vi "Set Multi.vi"(0 "Display State In":T2, 5 "Value":T1={"Active"=FALSE, "Delay (ms)"=0.0, "Duration (ms)"=50.0, "Ramp (ms)"=5.0, "Rate (Hz)"=0.0, "Trepeat (ms)"=0.0, "Repeat"=FALSE}, 7 "First":bool, 9 "Container State":T3, 11 "error in (no error)":errorcluster) -> (4 "Display State Out":T2, 15 "error out":errorcluster)   [LabVIEW 2015, in "Burst (G3).xctl"]
uses:
  Burst (G3).xctl
  <vilib>/_xctls/Container State.ctl
  State.ctl
  Utility VIs/Controls/KCheckbox/KCheckbox.xctl
  Utility VIs/Controls/KNumeric (DBL)/KNumeric (DBL).xctl
  Burst Data.ctl
  <vilib>/_xctls/XControlSupport.lvlib
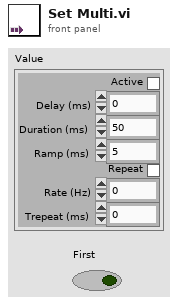
[diagram p1: front panel]
types:
  T1 = typedef "Burst (G3).xctl/Burst Data.ctl" = cluster{"Active":bool, "Delay (ms)":dbl, "Duration (ms)":dbl, "Ramp (ms)":dbl, "Rate (Hz)":dbl, "Trepeat (ms)":dbl, "Repeat":bool}
  T2 = typedef "Burst (G3).xctl/State.ctl" = cluster{"ctls":cluster{"Active":refnum<vi>, "Delay":refnum<vi>, "Dur":refnum<vi>, "Ramp":refnum<vi>, "Repeat":refnum<vi>, "at":refnum<vi>, "for":refnum<vi>}, "active mixed":bool, "repeat mixed":bool}
  T3 = typedef "XControlSupport.lvlib/Container State.ctl" = cluster{"Indicator?":bool, "Run Mode?":bool, " Refnum":refnum<vi>}
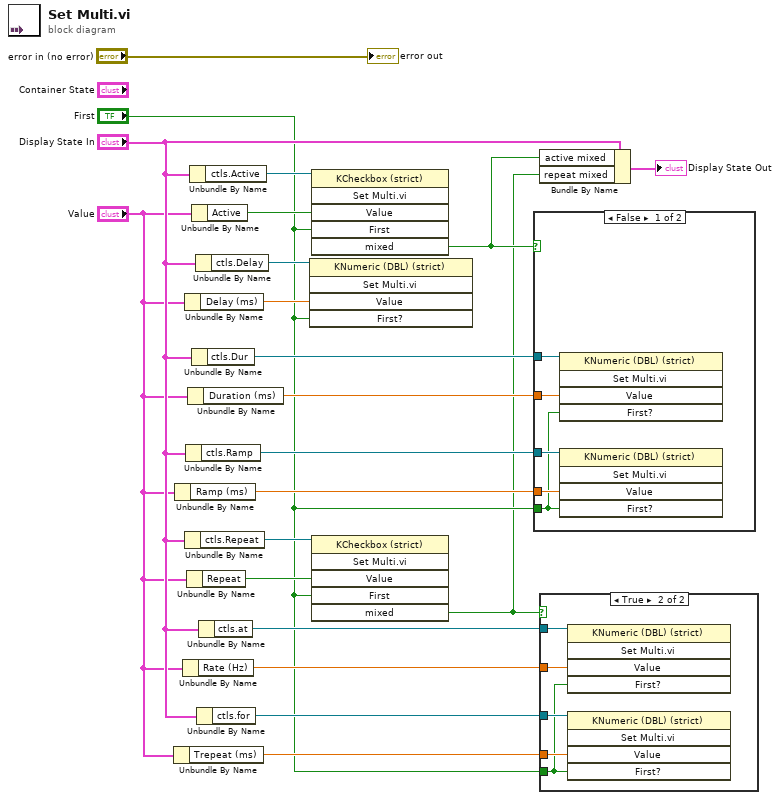
[diagram p0: block diagram]
diagram:
  n1 = Unbundle By Name("Value") -> ("Trepeat (ms)"=w10:dbl)
  n2 = Unbundle By Name("Value") -> ("Ramp (ms)"=w18:dbl)
  n3 = Unbundle By Name("Value") -> ("Rate (Hz)"=w16:dbl)
  n4 = Unbundle By Name("Value") -> ("Delay (ms)"=w5:dbl)
  n5 = Unbundle By Name("Display State In") -> ("ctls.Repeat"=w12:refnum<vi>)
  n6 = Unbundle By Name("Display State In") -> ("ctls.Ramp"=w13:refnum<vi>)
  n7 = Unbundle By Name("Value") -> ("Repeat"=w17:bool)
  n8 = Unbundle By Name("Value") -> ("Duration (ms)"=w14:dbl)
  n9 = Unbundle By Name("Display State In") -> ("ctls.Active"=w20:refnum<vi>)
  n10 = Unbundle By Name("Value") -> ("Active"=w19:bool)
  n11 = Unbundle By Name("Display State In") -> ("ctls.Dur"=w15:refnum<vi>)
  n12 = Unbundle By Name("Display State In") -> ("ctls.Delay"=w6:refnum<vi>)
  n13 = Unbundle By Name("Display State In") -> ("ctls.for"=w9:refnum<vi>)
  n14 = Unbundle By Name("Display State In") -> ("ctls.at"=w11:refnum<vi>)
  n15 = invoke class="KNumeric (DBL) (strict)" method="Set Multi.vi"(reference=w6, "Value"=w5, "First?"="First") -> ()  [unwired: 2 in, 5 out]
  n16 = invoke class="KCheckbox (strict)" method="Set Multi.vi"(reference=w20, "Value"=w19, "First"="First") -> ("mixed"=w2:bool)  [unwired: 3 in, 5 out]
  n17 = invoke class="KCheckbox (strict)" method="Set Multi.vi"(reference=w12, "Value"=w17, "First"="First") -> ("mixed"=w1:bool)  [unwired: 3 in, 5 out]
  n18 = case shown="False" w2 {
    tunnel: w18 -> [w26 _]
    tunnel: w15 -> [w25 _]
    tunnel: w14 -> [w24 _]
    tunnel: w13 -> [w23 _]
    tunnel: "First" -> [w22 _]
    frame False {
      n19 = invoke class="KNumeric (DBL) (strict)" method="Set Multi.vi"(reference=w25, "Value"=w24, "First?"=w22) -> ()  [unwired: 2 in, 5 out]
      n20 = invoke class="KNumeric (DBL) (strict)" method="Set Multi.vi"(reference=w23, "Value"=w26, "First?"=w22) -> ()  [unwired: 2 in, 5 out]
    }
    frame True {
    }
  }
  n21 = Bundle By Name(cluster="Display State In", "active mixed"=w2, "repeat mixed"=w1) -> (→"Display State Out":T2)
  n22 = case shown="True" w1 {
    tunnel: w16 -> [_ w31]
    tunnel: w11 -> [_ w30]
    tunnel: w10 -> [_ w29]
    tunnel: w9 -> [_ w28]
    tunnel: "First" -> [_ w27]
    frame False {
    }
    frame True {
      n23 = invoke class="KNumeric (DBL) (strict)" method="Set Multi.vi"(reference=w30, "Value"=w31, "First?"=w27) -> ()  [unwired: 2 in, 5 out]
      n24 = invoke class="KNumeric (DBL) (strict)" method="Set Multi.vi"(reference=w28, "Value"=w29, "First?"=w27) -> ()  [unwired: 2 in, 5 out]
    }
  }
  "error out" <- "error in (no error)"
